vi "CSMP-Async Call.vi"(0 "state":string, 1 "args":string, 2 "source/target":string, 5 "Error in":errorcluster caption="Error in (no error)", 8 "Module Name":string, 10 "Msg Type":T1) -> (14 "state out":string, 15 "args out":string, 16 "source/target out":string, 17 "Pre-State out":string, 18 "Pre-Args out":string, 19 "error":errorcluster)   [LabVIEW 2020, in "Communicable State Machine.lvlib"]
uses:
  Communicable State Machine.lvlib
  _CSM_MSG_TYPE.ctl
  _Cross CSM State Data.ctl
  _Cross CSM State Response.ctl
  _CSM_Response Source Message.ctl
  Priority Queue.lvclass/Priority Queue.ctl
  Enqueue Element.vi
  _CSMOFGV.vi
  CSM Not Allowed Message.vi
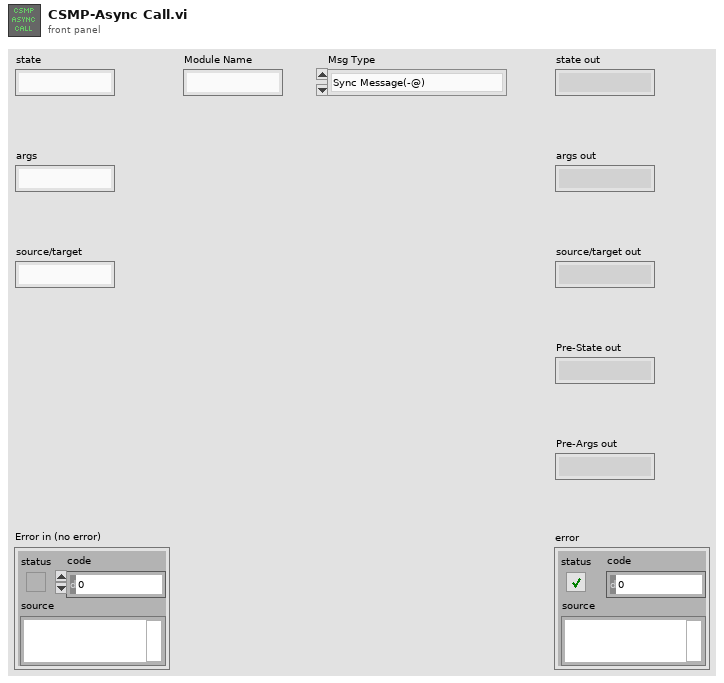
[diagram p1: front panel]
types:
  T1 = typedef "Communicable State Machine.lvlib/_CSM_MSG_TYPE.ctl" = enum16{"Sync Message(-@)", "Async Message(->)", "Async without Response(->|)", "Async Response", "Broadcast(-><all>)", "Broadcast(-><status>)", "Broadcast(-><interrupt>)", "Append to JKISM States", "Append to JKISM States(High Priority)"}
  T2 = typedef "Communicable State Machine.lvlib/_CSMObj.ctl" = cluster{"Requested Name":string, "Module Name":string, "Mode":T3, "Queue":refnum<class "Priority Queue.lvclass">, "CSM-Data":refnum<data-value>, "User Event":refnum<user-event>, "Status Change Event":refnum<user-event>, "Allowed Messages":string[], "Mode-Data":refnum<data-value>, "Group Name":string, "Exit Event":refnum<user-event>}
  T3 = typedef "Communicable State Machine.lvlib/_CSM_MODE.ctl" = enum16{"Not Exist", "Stand Alone", "CSM", "Worker Agent", "Worker", "Chain", "Chain Node"}
  T4 = typedef "Communicable State Machine.lvlib/_Cross CSM State Data.ctl" = cluster{"Msg Type":T1, "state":string, "args":string, "source":string, "RespQ":refnum<queue>, "Response For Message":T5, "Target":string}
  T5 = typedef "Communicable State Machine.lvlib/_CSM_Response Source Message.ctl" = cluster{"‘State":string, "’Arguments":string, "’Error":errorcluster}
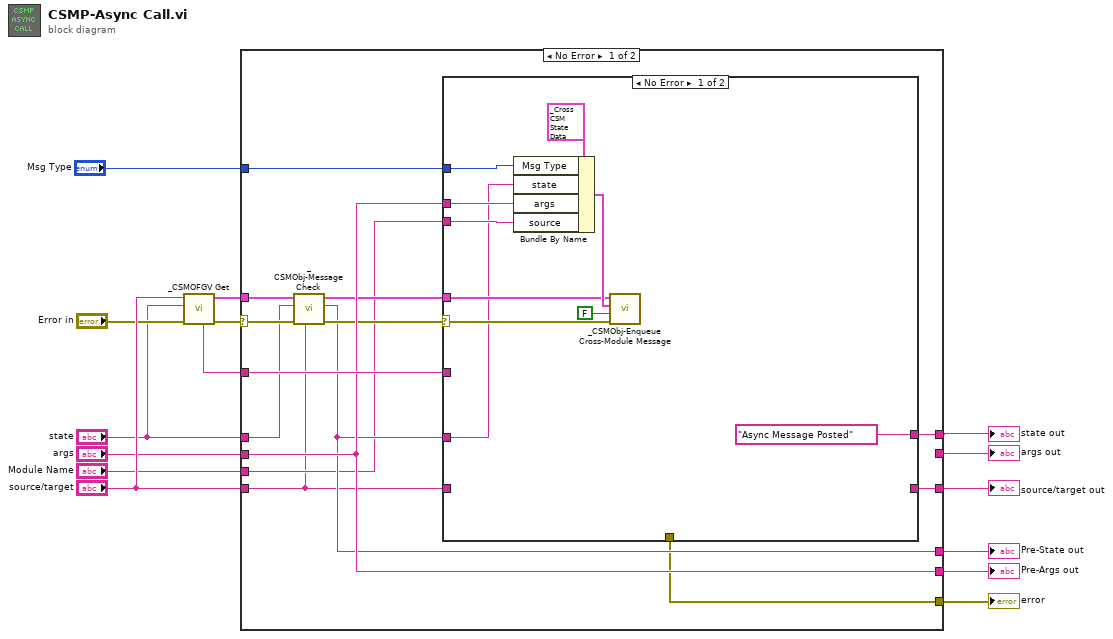
[diagram p0: block diagram]
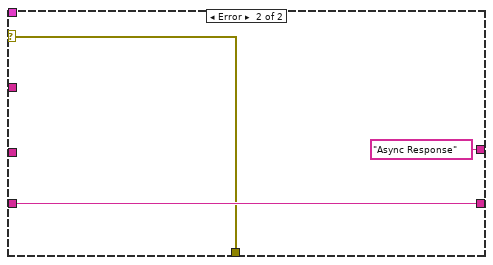
[diagram p2: hidden frame]
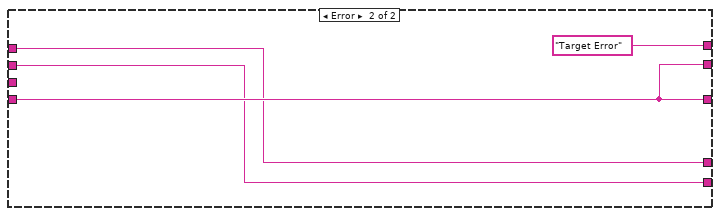
[diagram p3: hidden frame]
diagram:
  n1 = call "_CSMOFGV Get.vi"("Error in"="Error in", "Message"="state", "Name(\"\" to use uuid) in"="source/target") -> ("Error out"=w15:errorcluster, "CSM-Obj"=w13:T2, "Name"=w14:string)  [unwired: 6 in]
  n2 = case shown="No Error" w15 {
    selector: w15 -> [w23 _]
    tunnel: w13 -> [w24 _]
    tunnel: [w29 "Target Error" ("before match")] -> w9
    tunnel: [_ w45] -> w8
    tunnel: "source/target" -> [w16 w45]
    tunnel: "state" -> [w20 w44]
    tunnel: "args" -> [w26 w43]
    tunnel: "Module Name" -> [w17 _]
    tunnel: w14 -> [w28 _]
    tunnel: [w27 w45] -> w7
    tunnel: [w19 w44] -> w5
    tunnel: [w26 w43] -> w4
    tunnel: "Msg Type" -> [w25 _]
    tunnel: [w18 _] -> w2
    frame No Error {
      n3 = call "_CSMObj-Message Check.vi"("CSM"=w16, "Error in"=w23, "message"=w20, "CSMQ in"=w24) -> ("Error out"=w22:errorcluster, "message(dup)"=w19:string, "CSMQ out"=w21:T2)  [unwired: 5 in]
      n4 = case shown="No Error" w22 {
        selector: w22 -> [w32 w40]
        tunnel: w17 -> [w38 _]
        tunnel: ["Async Message Posted" ("before match") "Async Response" ("f")] -> w29
        tunnel: w28 -> [_ _]
        tunnel: w16 -> [_ w42]
        tunnel: [_ w42] -> w27
        tunnel: w26 -> [w34 _]
        tunnel: w25 -> [w33 _]
        tunnel: w21 -> [w31 _]
        tunnel: w19 -> [w30 _]
        tunnel: [_ w40] -> w18
        frame No Error {
          n5 = Bundle By Name(cluster=T4 {"Msg Type"=enum."Sync Message(-@)", "state"="", "args"="", "source"="", "RespQ"=refnum, "Response For Message"={"‘State"="", "’Arguments"="", "’Error"={"status"=FALSE, "code"=0, "source"=""}}, "Target"=""} ("Cross JKI State Machine State"), "Msg Type"=w33, "state"=w30, "args"=w34, "source"=w38) -> (w37:T4)
          n6 = call "_CSMObj-Enqueue Cross-Module Message.vi"("Error in"=w32, "High Priority?(F)"=FALSE, "Data"=w37, "CSMQ in"=w31) -> ()  [unwired: 6 in, 2 out]
        }
        frame Error {
        }
      }
    }
    frame Error {
    }
  }
  "state out" <- w9
  "args out" <- w8
  "source/target out" <- w7
  "Pre-State out" <- w5
  "Pre-Args out" <- w4
  "error" <- w2
